vi "GetCaseFrameByName.vi"(8 "error in (no error)":errorcluster, 10 "FrameName":string, 11 "CaseStructure Ref":refnum<vi>) -> (0 "error out":errorcluster, 2 "Frame Ref":refnum<vi>, 3 "CaseStructure Ref":refnum<vi>)   [LabVIEW 2019, in "BlueUtilityScripts.lvlib"]
uses:
  BlueUtilityScripts.lvlib
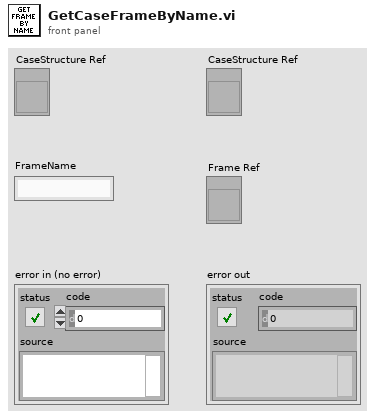
[diagram p1: front panel]
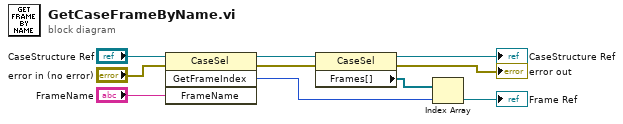
[diagram p0: block diagram]
diagram:
  n1 = invoke class="CaseSel" method="GetFrameIndex"(reference="CaseStructure Ref", error in="error in (no error)", "FrameName"="FrameName") -> (reference out=w4:refnum<vi>, error out=w3:errorcluster, "GetFrameIndex"=w2:i32)  [unwired: 1 in, 1 out]
  n2 = property class="CaseSel"(reference=w4, error in=w3) -> (reference out=→"CaseStructure Ref":refnum<vi>, error out=→"error out":errorcluster, "Frames[]"=w5:refnum<vi>[])
  n3 = Index Array(array=w5, index=w2) -> (element=→"Frame Ref":refnum<vi>)
